vi "ni5660 Read IQ.vi"(0 "receiver info in":T1, 5 "timeout (sec)":dbl=5.0 format="%.2f", 11 "error in (no error)":errorcluster) -> (4 "receiver info out":T1, 6 "IQ waveform":cluster{"t0":dbl, "dt":dbl, "Y":cdb[]} {"Y" format="%.2g"; "dt" format="%.2g"; "t0" format="%.2g"}, 15 "error out":errorcluster)   [LabVIEW 2011]
doc: "This VI returns the waveform acquired by the RF Signal Analyzer. This VI initiates an acquisition and returns both a scaled voltage waveform with timing information, and IQ data computed through a process of filtering, decimation, and downconversion."
uses:
  <vilib>/addons/Modulation/niScope/controls/mod_Modulation Settings.ctl
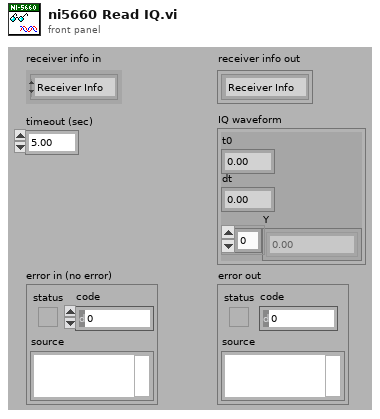
[diagram p1: front panel]
types:
  T1 = typedef "mod_Modulation Settings.ctl" = cluster{enum16{"Receiver Info"}, variant}
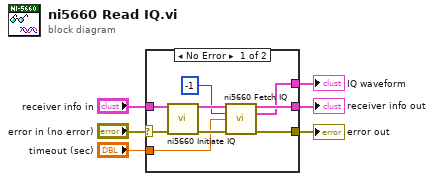
[diagram p0: block diagram]
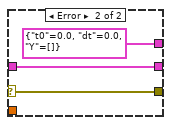
[diagram p2: hidden frame]
diagram:
  n1 = case shown="No Error" "error in (no error)" {
    selector: "error in (no error)" -> [w13 w18]
    tunnel: [w15 w18] -> w6
    tunnel: "receiver info in" -> [w12 w17]
    tunnel: [w14 w17] -> w3
    tunnel: "timeout (sec)" -> [w8 _]
    tunnel: [w7 cluster{"t0":dbl, "dt":dbl, "Y":cdb[]} {"t0"=0.0, "dt"=0.0, "Y"=[]} ("IQ data (complex)")] -> w1
    frame No Error {
      n2 = call <instrlib>:"ni5660 Initiate IQ.vi"("receiver info in"=w12, "error in (no error)"=w13) -> ("receiver info out"=w11:T1, "error out"=w10:errorcluster)  [unwired: 12 in]
      n3 = call <instrlib>:"ni5660 Fetch IQ.vi"("receiver info in"=w11, "samples to read"=-1, "timeout (sec)"=w8, "error in (no error)"=w10) -> ("receiver info out"=w14:T1, "IQ waveform"=w7:cluster{"t0":dbl, "dt":dbl, "Y":cdb[]}, "error out"=w15:errorcluster)  [unwired: 9 in]
    }
    frame Error {
    }
  }
  "error out" <- w6
  "receiver info out" <- w3
  "IQ waveform" <- w1
